vi "MeasSingleVoltCont.vi"   [LabVIEW 2014]
uses:
  Controls/measVoltState.ctl
  <vilib>/Platform/TimedLoop/XDataNode/timing_clust.ctl
  <vilib>/Platform/TimedLoop/XDataNode/nitl_modes.ctl
  <vilib>/Platform/TimedLoop/XDataNode/wakeup.ctl
  <vilib>/rvi/Emulation/niFpgaGetClockAttributes.vi
  <vilib>/rvi/Emulation/niFpgaSctlEmulationGetInTimedLoop.vi
  <vilib>/rvi/Emulation/niFpgaEmulationReportErrorSimple.vi
  <vilib>/rvi/Emulation/niFpgaCriticalErrorInLSC.vi
  <vilib>/rvi/Emulation/niFpgaEmulationIsFPGAContextNoSignature.vi
  <vilib>/rvi/DataTransferAndStorage/Container/Common/niFpgaContainerGetUniqueNameForEmu.vi
  <vilib>/rvi/eio/common/nirviEmuReportErrorAndStop.vi
  <vilib>/rvi/Emulation/niFpgaProcessEmulError.vi
  measVoltGlobVars.vi
  <vilib>/rvi/eio/common/nirviEmuTemplateMethod_errors.vi
  <vilib>/Platform/TimedLoop/XDataNode/XDataNode.xnode
  <vilib>/rvi/DataTransferAndStorage/Container/XNode/niFpgaContainer.xnode
  <vilib>/rvi/DataTransferAndStorage/Handshake/Emulation/niFpgaHandshakeEmulation.vi
  <vilib>/eio/EIONode/EIONode.xnode
  <vilib>/Platform/TimedLoop/XDataNode/XDNodeRunTimeDep.lvlib
types:
  T1 = typedef "measVoltState.ctl" = enum16{"Idle", "sendMeasRequest", "waitUntilDone", "done"}
  T2 = typedef "XDNodeRunTimeDep.lvlib/timing_clust.ctl" = cluster{"Expected End [f-1]":u64, "Actual End [f-1]":u64, "Finished Late? [f-1]":bool, "Expected End [i-1]":u64, "Actual End [i-1]":u64, "Finished Late? [i-1]":bool, "Expected Start [i]":u64, "Actual Start [i]":u64, "Expected Start [f]":u64, "Actual Start [f]":u64, "Source Name":string, "Structure Name":string, "Period":i64, "Deadline":i64, "Offset":i64, "Start":i64, "Priority":i32, "Timeout":i32, "Mode":T3, "Wakeup Reason":T4, "Error":errorcluster, "Source Type":string, "Secondary Source Type":string, "Global End Time":u64, "Global Start Time":u64, "Frame Duration":u64, "Iteration Duration":u64, "Assigned CPU":i32, "I/O Scan Engine Mode":u32}
  T3 = typedef "XDNodeRunTimeDep.lvlib/nitl_modes.ctl" = enum32{"No Change", "Process missed periods, maintain original phase", "Discard missed periods, maintain original phase", "Process missed periods, ignore original phase", "Discard missed periods, ignore original phase"}
  T4 = typedef "XDNodeRunTimeDep.lvlib/wakeup.ctl" = enum32{"Normal", "Aborted", "Asynchronous wakeup", "Timing source error", "Timed loop error", "Timeout"}
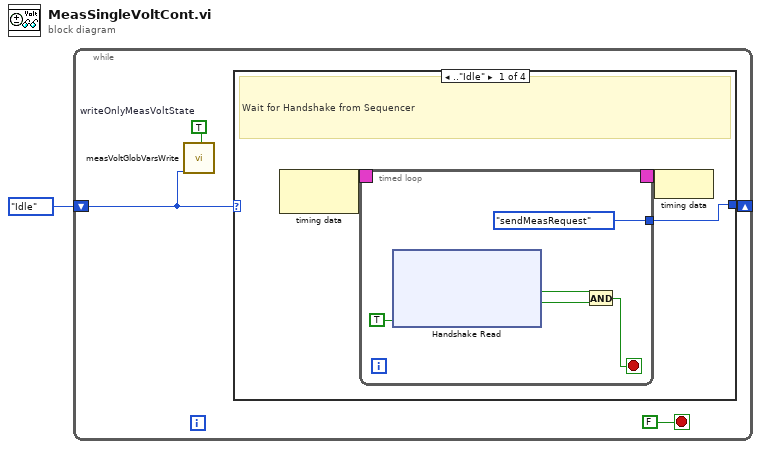
[diagram p0: block diagram]
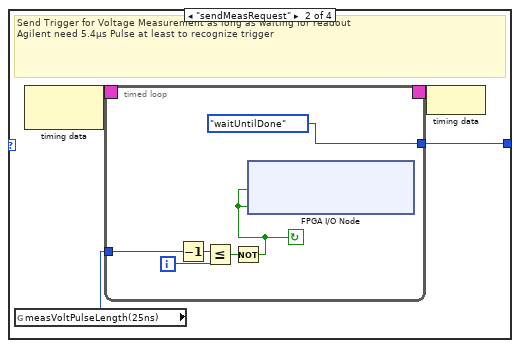
[diagram p2: hidden frame]
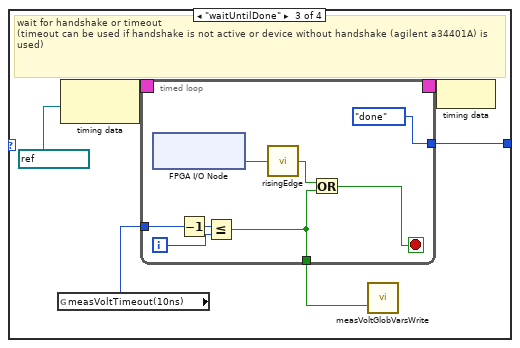
[diagram p3: hidden frame]
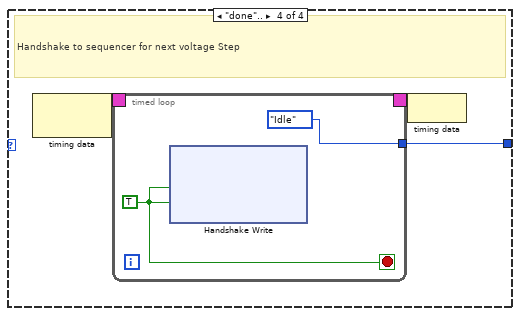
[diagram p4: hidden frame]
diagram:
  n1 = while {
    shift-right: [w4] -> _
    shift-left: measVoltState."Idle" ("measVoltState") -> [w3]
    stop <- FALSE stop-if-true
    w2 = TRUE  # writeOnlyMeasVoltState
    n2 = call "measVoltGlobVarsWrite.vi"("measVoltState"=w3, "writeOnlyMeasVoltState"=w2) -> ()  [unwired: 18 in]
    n3 = case shown="..\"Idle\"" w3 {
      tunnel: [w6 w18 w33 w52] -> w4
      frame .."Idle" {
        # "Wait for Handshake from Sequencer"
        n4 = node-c288() -> (w8:T2)  [unwired: 1 in]
        n5 = timed-loop {
          timing: w8 -> [_]
          timing-out: [_] -> w7
          tunnel: [measVoltState."sendMeasRequest" ("measVoltState")] -> w6
          stop <- w10 stop-if-true
          n6 = xnode ("Handshake Read")("Ready for Output"=TRUE) -> ("Data"=w12:bool, "Output Valid"=w11:bool)  [unwired: 1 in, 1 out]
          n7 = And(x=w12, y=w11) -> (x .and. y?=w10:bool)
        }
        n8 = node-c288(w7) -> ()
      }
      frame "sendMeasRequest" {
        # "Send Trigger for Voltage Measurement as long as waiting for readout\nAgilent need 5.4µs Pulse at least to recognize trigger"
        n9 = global read "measVoltGlobVars.vi" "measVoltPulseLength(25ns)"() -> (w19:i32)
        n10 = node-c288() -> (w21:T2)  [unwired: 1 in]
        n11 = timed-loop {
          timing: w21 -> [_]
          timing-out: [_] -> w20
          tunnel: w19 -> [w23]
          tunnel: [measVoltState."waitUntilDone" ("measVoltState")] -> w18
          i -> [w27]
          stop <- w24 continue-if-true
          n12 = Decrement(x=w23) -> (x-1=w26:i32)
          n13 = Less Or Equal?(x=w26, y=w27) -> (x <= y?=w25:bool)
          n14 = Not(x=w25) -> (.not. x?=w24:bool)
          n15 = xnode "FPGA I/O Node"("PXI_Trig3"=w24, "measVoltFlagDio8Con1"=w24) -> ()  [unwired: 2 in, 2 out]
        }
        n16 = node-c288(w20) -> ()
      }
      frame "waitUntilDone" {
        # "wait for handshake or timeout \n(timeout can be used if handshake is not active or device without handshake (agilent a34401A) is used)"
        n17 = global read "measVoltGlobVars.vi" "measVoltTimeout(10ns)"() -> (w35:i32)
        n18 = node-c288(refnum<k21> "100MHz" ("Source Name")) -> (w37:T2)
        n19 = timed-loop {
          timing: w37 -> [_]
          timing-out: [_] -> w36
          tunnel: w35 -> [w44]
          tunnel: [w39] -> w34
          tunnel: [measVoltState."done" ("measVoltState")] -> w33
          i -> [w43]
          stop <- w42 stop-if-true
          n20 = xnode "FPGA I/O Node"() -> ("PXI_Trig4"=w41:bool)  [unwired: 1 in, 1 out]
          n21 = Decrement(x=w44) -> (x-1=w45:i32)
          n22 = Less Or Equal?(x=w45, y=w43) -> (x <= y?=w39:bool)
          n23 = call "risingEdge.vi"("In"=w41) -> ("out"=w40:bool)
          n24 = Or(x=w40, y=w39) -> (x .or. y?=w42:bool)
        }
        n25 = call "measVoltGlobVarsWrite.vi"("timedOutWhileHandshake"=w34) -> ()  [unwired: 19 in]
        n26 = node-c288(w36) -> ()
      }
      frame "done".. {
        # "Handshake to sequencer for next voltage Step"
        n27 = node-c288() -> (w54:T2)  [unwired: 1 in]
        n28 = timed-loop {
          timing: w54 -> [_]
          timing-out: [_] -> w53
          tunnel: [measVoltState."Idle" ("measVoltState")] -> w52
          stop <- w56 stop-if-true
          w56 = TRUE ("Ready for Output")
          n29 = xnode ("Handshake Write")("Data"=w56, "Input Valid"=w56) -> ()  [unwired: 1 in, 2 out]
        }
        n30 = node-c288(w53) -> ()
      }
    }
  }
